vi "TPD.vi"(0 "Input":dbl, 1 "reset":bool, 2 "Tol":dbl step=0.01) -> (3 "Global Hi Peak":dbl, 4 "Global Lo Peak":dbl, 6 "Up ?":bool, 7 "Up ?":i64, 8 "Local Hi Peak":dbl, 9 "Local Lo Peak":dbl)   [LabVIEW 2011]
panel:
  out "Dn Test":bool
  out "Up Test":bool
  out "Prev Lo Pk":dbl
  out "Prev Hi Pk":dbl
  out "Prev Dir":bool
  out "Lo Tol":dbl
  out "Hi Tol":dbl
  out "Waveform Chart":cluster{dbl, dbl, dbl, dbl, dbl}(graph)
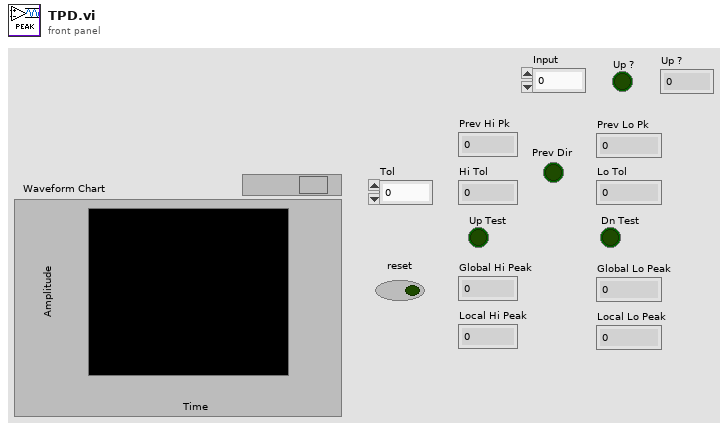
[diagram p1: front panel]
types:
  T1 = cluster{"Input":dbl, "Input":dbl, "Input":dbl, "Input":dbl, "Input":dbl}
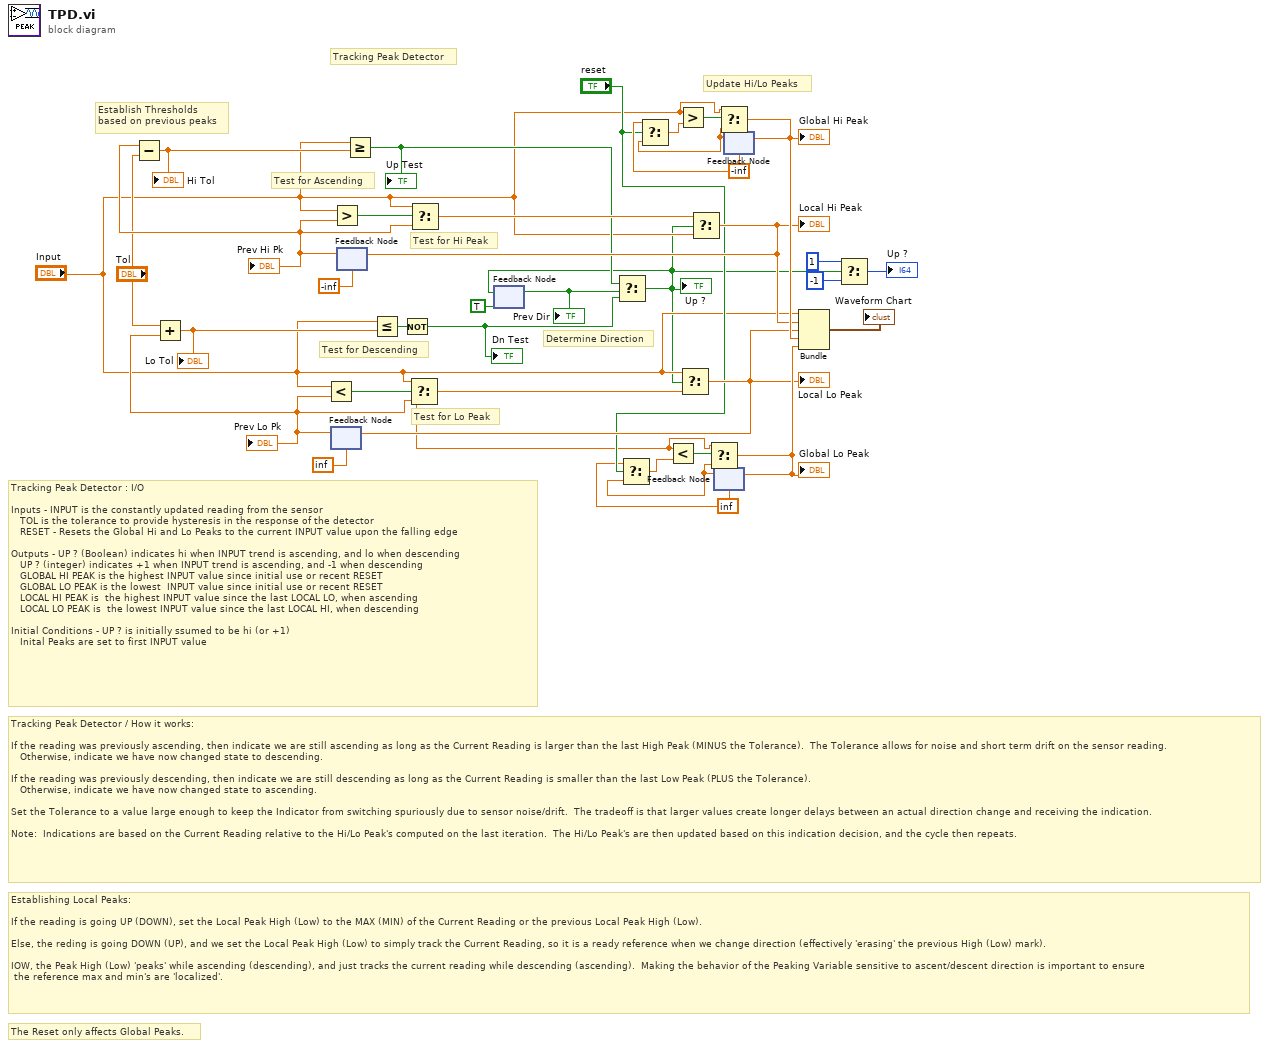
[diagram p0: block diagram]
diagram:
  w8 = inf
  w12 = -inf
  # "Tracking Peak Detector : I/O\n\nInputs - INPUT is the constantly updated reading from the sensor\n   TOL is the tolerance to provide hysteresis in the response of the detector\n   RESET - Resets the Global Hi and Lo Peaks to the current INPUT value upon the falling edge \n\nOutputs - UP ? (Boolean) indicates hi when INPUT trend is ascending, and lo when descending\n   UP ? (integer) indicates +1 when INPUT trend is ascending, and -1 when descending\n   GLOBAL HI PEAK is the highest INPUT value since initial use or recent RESET\n   GLOBAL LO PEAK is the lowest  INPUT value since initial use or recent RESET\n   LOCAL HI PEAK is  the highest INPUT value since the last LOCAL LO, when ascending\n   LOCAL LO PEAK is  the lowest INPUT value since the last LOCAL HI, when descending\n\nInitial Conditions - UP ? is initially ssumed to be hi (or +1)\n   Inital Peaks are set to first INPUT value"
  # "The Reset only affects Global Peaks."
  # "Establishing Local Peaks:\n\nIf the reading is going UP (DOWN), set the Local Peak High (Low) to the MAX (MIN) of the Current Reading or the previous Local Peak High (Low).\n\nElse, the reding is going DOWN (UP), and we set the Local Peak High (Low) to simply track the Current Reading, so it is a ready reference when we change direction (effectively 'erasing' the previous High (Low) mark).\n\nIOW, the Peak High (Low) 'peaks' while ascending (descending), and just tracks the current reading while descending (ascending).  Making the behavior of the Peaking Variable sensitive to ascent/descent direction is important to ensure\n the reference max and min's are 'localized'."
  # "Tracking Peak Detector / How it works:\n\nIf the reading was previously ascending, then indicate we are still ascending as long as the Current Reading is larger than the last High Peak (MINUS the Tolerance).  The Tolerance allows for noise and short term drift on the sensor reading.\n   Otherwise, indicate we have now changed state to descending.\n\nIf the reading was previously descending, then indicate we are still descending as long as the Current Reading is smaller than the last Low Peak (PLUS the Tolerance).\n   Otherwise, indicate we have now changed state to ascending.\n\nSet the Tolerance to a value large enough to keep the Indicator from switching spuriously due to sensor noise/drift.  The tradeoff is that larger values create longer delays between an actual direction change and receiving the indication.\n\nNote:  Indications are based on the Current Reading relative to the Hi/Lo Peak's computed on the last iteration.  The Hi/Lo Peak's are then updated based on this indication decision, and the cycle then repeats."
  # "Determine Direction"
  # "Update Hi/Lo Peaks"
  # "Test for Ascending"
  # "Test for Descending"
  # "Test for Lo Peak"
  # "Test for Hi Peak"
  # "Establish Thresholds\nbased on previous peaks"
  # "Tracking Peak Detector"
  n1 = feedback #1(inf) -> (w20:dbl)
  "Prev Lo Pk" <- w20
  n2 = Add(x="Tol", y=w20) -> (x+y=w27:dbl)
  "Lo Tol" <- w27
  n3 = Less?(x="Input", y=w20) -> (x < y?=w33:bool)
  n4 = feedback #2(-inf) -> (w26:dbl)
  "Prev Hi Pk" <- w26
  n5 = Subtract(x=w26, y="Tol") -> (x-y=w28:dbl)
  "Hi Tol" <- w28
  n6 = Greater?(x="Input", y=w26) -> (0:w34:bool)
  n7 = Greater Or Equal?(x="Input", y=w28) -> (x >= y?=w6:bool)
  "Up Test" <- w6
  n8 = Less Or Equal?(x="Input", y=w27) -> (x <= y?=w23:bool)
  n9 = Not(x=w23) -> (.not. x?=w22:bool)
  "Dn Test" <- w22
  n10 = Select(t="Input", s=w33, f=w20) -> (s? t:f=w24:dbl)
  n11 = Select(t="Input", s=w34, f=w26) -> (s? t:f=w25:dbl)
  n12 = feedback #3(TRUE) -> (w29:bool)
  "Prev Dir" <- w29
  n13 = Select(t=w6, s=w29, f=w22) -> (s? t:f=w2:bool)
  "Up ?" <- w2
  n14 = feedback-in #3(w2) -> ()
  n15 = Select(t="Input", s=w2, f=w24) -> (s? t:f=w16:dbl)
  "Local Lo Peak" <- w16
  n16 = feedback-in #1(w16) -> ()
  n17 = Select(t=w25, s=w2, f="Input") -> (s? t:f=w15:dbl)
  "Local Hi Peak" <- w15
  n18 = feedback-in #2(w15) -> ()
  n19 = feedback #4(w8) -> (w9:dbl)
  n20 = Select(t=w8, s="reset", f=w9) -> (s? t:f=w11:dbl)
  n21 = Less?(x="Input", y=w11) -> (x < y?=w19:bool)
  n22 = Select(t="Input", s=w19, f=w9) -> (s? t:f=w17:dbl)
  "Global Lo Peak" <- w17
  n23 = feedback-in #4(w17) -> ()
  n24 = feedback #5(w12) -> (w14:dbl)
  n25 = Select(t=w12, s="reset", f=w14) -> (s? t:f=w13:dbl)
  n26 = Greater?(x="Input", y=w13) -> (0:w7:bool)
  n27 = Select(t="Input", s=w7, f=w14) -> (s? t:f=w18:dbl)
  "Global Hi Peak" <- w18
  n28 = feedback-in #5(w18) -> ()
  n29 = Bundle("Input"="Input", "Input"=w15, "Input"=w16, "Input"=w18, "Input"=w17) -> (→"Waveform Chart":T1)  [unwired: 1 in]
  n30 = Select(t=i64 1, s=w2, f=i64 -1) -> (s? t:f=→"Up ?":i64)
